vi "Write Origin.vi"(8 "error in (no error)":errorcluster, 10 "Origin":T1, 11 "SubPanel.lvclass in":refnum<class "SubPanel.lvclass">) -> (0 "error out":errorcluster, 3 "SubPanel.lvclass out":refnum<class "SubPanel.lvclass">)   [LabVIEW 2015, in "SubPanel.lvclass"]
uses:
  SubPanel.lvclass
  <vilib>/Utility/miscctls.llb/LVPointTypeDef.ctl
  SubPanel.lvclass/SubPanel.ctl
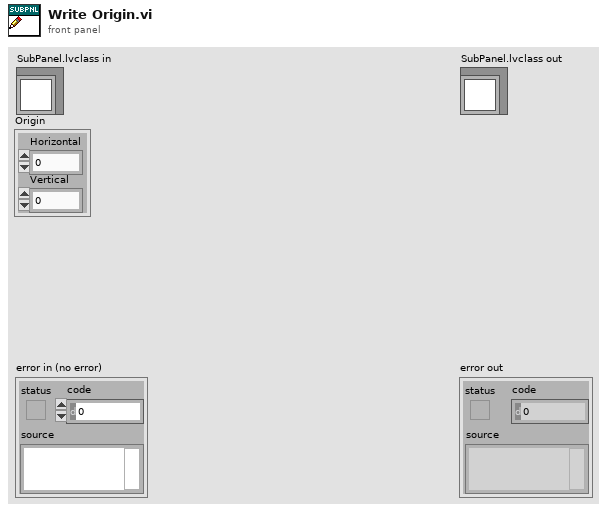
[diagram p1: front panel]
types:
  T1 = typedef "LVPointTypeDef.ctl" = cluster{"Horizontal":i16, "Vertical":i16}
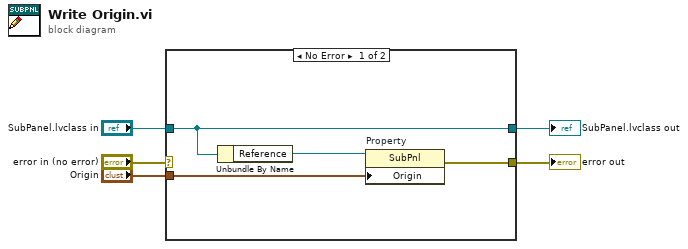
[diagram p0: block diagram]
diagram:
  n1 = case shown="No Error" "error in (no error)" {
    selector: "error in (no error)" -> [_ w11]
    tunnel: [w9 w11] -> w4
    tunnel: [w7 w10] -> w2
    tunnel: "SubPanel.lvclass in" -> [w7 w10]
    tunnel: "Origin" -> [w8 _]
    frame No Error {
      n2 = Unbundle By Name(w7) -> ("Reference"=w6:refnum<vi>)
      n3 = property on="Property" class="SubPnl"(reference=w6, "Origin"=w8) -> (error out=w9:errorcluster)  [unwired: 1 in, 1 out]
    }
    frame Error {
    }
  }
  "error out" <- w4
  "SubPanel.lvclass out" <- w2
